vi "Write CurrentChannel.vi"(8 "error in (no error)":errorcluster, 10 "CurrentChannel":string="CHAN1", 11 "Agilent DSO-X 3032A in":refnum<class "Agilent DSO-X 3032A.lvclass">) -> (0 "error out":errorcluster, 3 "Agilent DSO-X 3032A out":refnum<class "Agilent DSO-X 3032A.lvclass">)   [LabVIEW 2014, in "Agilent DSO-X 3032A.lvclass"]
uses:
  Agilent DSO-X 3032A.lvclass
  Agilent DSO-X 3032A.lvclass/Agilent DSO-X 3032A.ctl
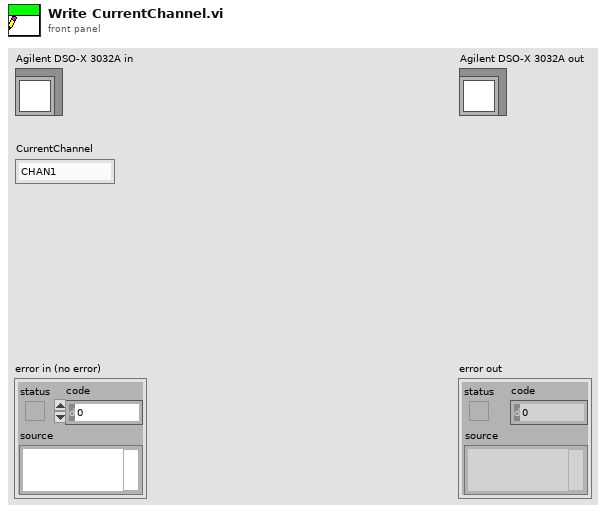
[diagram p1: front panel]
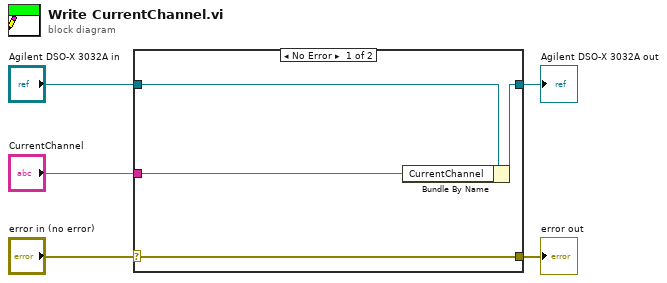
[diagram p0: block diagram]
diagram:
  n1 = case shown="No Error" "error in (no error)" {
    selector: "error in (no error)" -> [w9 w10]
    tunnel: [w9 w10] -> w4
    tunnel: [w7 w11] -> w2
    tunnel: "Agilent DSO-X 3032A in" -> [w8 w11]
    tunnel: "CurrentChannel" -> [w6 _]
    frame No Error {
      n2 = Bundle By Name(cluster=w8, "CurrentChannel"=w6) -> (w7:refnum<class "Agilent DSO-X 3032A.lvclass">)
    }
    frame Error {
    }
  }
  "error out" <- w4
  "Agilent DSO-X 3032A out" <- w2
